vi "Lang.translate.vi"(8 "error in (no error)":errorcluster caption="错误输入（无错误）", 9 "key":string caption="密钥", 10 "lang":enum16{"zh", "en", "it"}(ring), 11 "基路径":path) -> (0 "error out":errorcluster caption="错误输出", 2 "value":string caption="值", 3 "Find?":bool)   [LabVIEW 2012, in "Lib_UEL.ATE.lvlib" / "Lib_App.lvlib"]
uses:
  <vilib>/Utility/config.llb/Read Key (String).vi
  Lib_App.lvlib
  <vilib>/Utility/config.llb/NI_LVConfig.lvlib
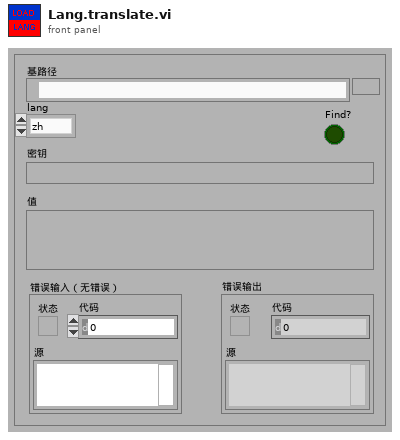
[diagram p1: front panel]
types:
  T1 = typedef "NI_LVConfig.lvlib/Config Data RefNum.ctl" = refnum<k1>
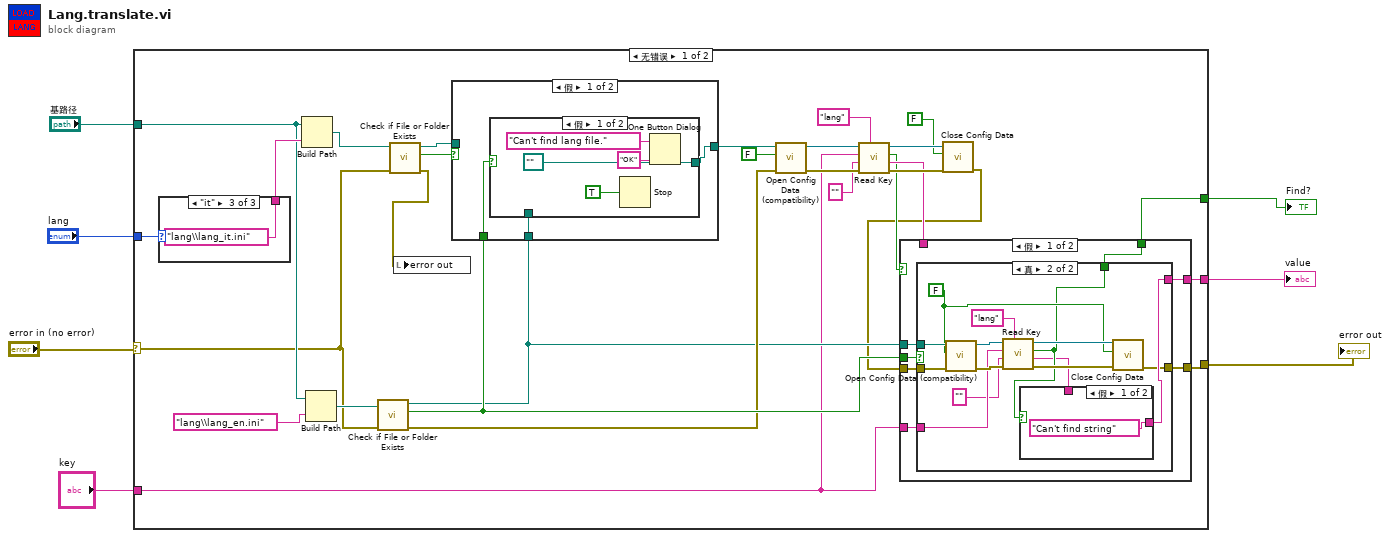
[diagram p0: block diagram]
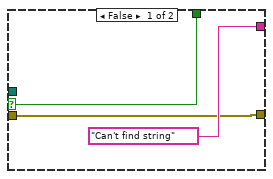
[diagram p2: hidden frame]
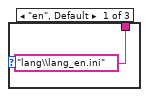
[diagram p7: hidden frame]
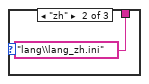
[diagram p8: hidden frame]
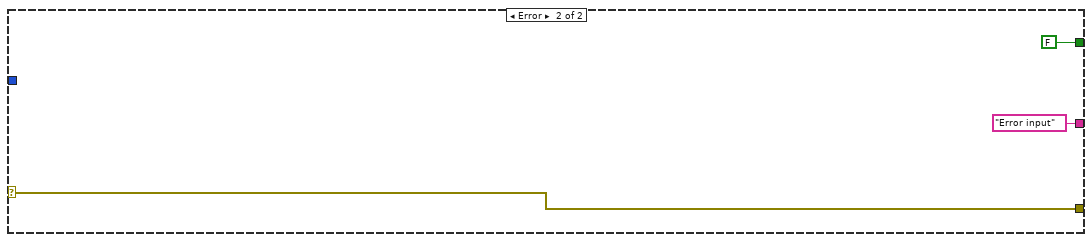
[diagram p9: hidden frame]
diagram:
  n1 = case shown="无错误" "error in (no error)" {
    selector: "error in (no error)" -> [w29 w80]
    tunnel: "基路径" -> [w32 _]
    tunnel: "lang" -> [w35 _]
    tunnel: [w8 w80] -> w4
    tunnel: "key" -> [w11 _]
    tunnel: [w17 "Error input" ("value")] -> w2
    tunnel: [w10 FALSE ("found?")] -> w1
    frame No Error {
      n2 = case shown="\"it\"" w35 {
        tunnel: ["lang\\lang_en.ini" ("名称或相对路径") "lang\\lang_zh.ini" ("名称或相对路径") "lang\\lang_it.ini" ("名称或相对路径")] -> w36
        frame "en", Default {
        }
        frame "zh" {
        }
        frame "it" {
        }
      }
      n3 = Build Path(base path=w32, name or relative path=w36) -> (appended path=w34:path)
      n4 = Build Path(base path=w32, name or relative path="lang\\lang_en.ini" ("名称或相对路径")) -> (appended path=w30:path)
      n5 = call <vilib>:"Check if File or Folder Exists.vi"("error in (no error)"=w29, "path"=w30) -> ("error out"=w13:errorcluster, "file or folder exists?"=w14:bool, "dup path"=w12:path)  [unwired: 7 in]
      n6 = call <vilib>:"Check if File or Folder Exists.vi"("error in (no error)"=w29, "path"=w34) -> ("error out"=w27:errorcluster, "file or folder exists?"=w33:bool, "dup path"=w28:path)  [unwired: 7 in]
      n7 = local write "error out"(w27) -> ()
      n8 = case shown="假" w33 {
        tunnel: [w67 w74] -> w26
        tunnel: w28 -> [_ w74]
        tunnel: w14 -> [w68 _]
        tunnel: w12 -> [w66 _]
        frame False {
          n9 = case shown="假" w68 {
            tunnel: [path "" ("dup path") w73] -> w67
            tunnel: w66 -> [_ w73]
            frame False {
              n10 = Stop(stop? (T)=TRUE ("停止？(T)")) -> ()
              n11 = One Button Dialog(message="Can't find lang file." ("消息"), button name ("OK")="OK" ("按钮名称（“确定”）")) -> ()  [unwired: 1 out]
            }
            frame True {
            }
          }
        }
        frame True {
        }
      }
      n12 = call <vilib>:"Open Config Data (compatibility).vi"("error in (no error)"=w13, "create file if necessary (T)"=FALSE ("create file if necessary? (T)"), "configuration file path"=w26) -> ("error out"=w23:errorcluster, "refnum"=w24:T1)  [unwired: 6 in, 1 out]
      n13 = call-poly <vilib>:"Read Key.vi"("section"="lang", "error in (no error)"=w23, "default value"="" ("section"), "key"=w11, "refnum"=w24) -> ("error out"=w19:errorcluster, "value"=w18:string, "found?"=w15:bool, "refnum out"=w20:T1)  [unwired: 3 in]
      n14 = call <vilib>:"Close Config Data.vi"("error in (no error)"=w19, "write file if changed (T)"=FALSE ("write configuration file? (T)"), "refnum"=w20) -> ("error out"=w9:errorcluster)  [unwired: 7 in, 1 out]
      n15 = case shown="假" w15 {
        selector: w15 -> [_ w64]
        tunnel: w18 -> [_ w65]
        tunnel: [w43 w65] -> w17
        tunnel: w14 -> [w42 _]
        tunnel: w9 -> [w41 w63]
        tunnel: w12 -> [w40 _]
        tunnel: w11 -> [w39 _]
        tunnel: [w38 w64] -> w10
        tunnel: [w37 w63] -> w8
        frame False {
          n16 = case shown="真" w42 {
            selector: w42 -> [w45 _]
            tunnel: ["Can't find string" ("value") w50] -> w43
            tunnel: w41 -> [w44 w56]
            tunnel: w40 -> [_ w55]
            tunnel: w39 -> [_ w54]
            tunnel: [w45 w51] -> w38
            tunnel: [w44 w47] -> w37
            frame False {
            }
            frame True {
              w52 = FALSE ("create file if necessary? (T)")
              n17 = call <vilib>:"Open Config Data (compatibility).vi"("error in (no error)"=w56, "create file if necessary (T)"=w52, "configuration file path"=w55) -> ("error out"=w58:errorcluster, "refnum"=w57:T1)  [unwired: 6 in, 1 out]
              n18 = call-poly <vilib>:"Read Key.vi"("section"="lang", "error in (no error)"=w58, "default value"="" ("section"), "key"=w54, "refnum"=w57) -> ("error out"=w60:errorcluster, "value"=w49:string, "found?"=w51:bool, "refnum out"=w59:T1)  [unwired: 3 in]
              n19 = case shown="假" w51 {
                tunnel: ["Can't find string" ("value") w62] -> w50
                tunnel: w49 -> [_ w62]
                frame False {
                }
                frame True {
                }
              }
              n20 = call <vilib>:"Close Config Data.vi"("error in (no error)"=w60, "write file if changed (T)"=w52, "refnum"=w59) -> ("error out"=w47:errorcluster)  [unwired: 7 in, 1 out]
            }
          }
        }
        frame True {
        }
      }
    }
    frame Error {
    }
  }
  "error out" <- w4
  "value" <- w2
  "Find?" <- w1
